vi "GageDeepAcquisition_ori.vi"() -> ()   [LabVIEW 2013]
uses:
  <vilib>/Analysis/NI_AALPro.lvlib
  <vilib>/Analysis/NI_AALBase.lvlib
  <vilib>/Utility/file.llb/Write To Spreadsheet File (DBL).vi
  <vilib>/Analysis/2dsp.llb/1D Cross Correlation (DBL).vi
panel:
  in  "하위 컷오프(MHz)":dbl
  in  "상위 컷오프(MHz)":dbl
  in  "시작":bool
  in  "Boolean":bool
  out "Path":path
  out "?":dbl[](graph)
  out "?":dbl[](graph)
  out "진행상황":string
  in  "crosscorr lacks":dbl=500.0
  out "Length":dbl=25000064.0
  out "?":dbl[](graph)
  in  "Trigger":T1={"Slope"=0, "Level"=0, "Source"=0, "External Range"=2000, "External Coupling"=0, "External"=FALSE, "Disable"=FALSE, "External Impedance"=1} {"External Impedance" items=["50 Ohm", "HiZ"]; "External Coupling" items=["DC", "AC"]; "External Range" min=2000 max=10000 step=8000; "Slope" items=["Rising", "Falling"]; "Level" min=-100 max=100; "Source" min=0 max=64 step=1}
  in  "stop":bool
  out "Page Size":dbl=98304.0 min=4096.0 step=4096.0
  out "Status":string
  in  "Channels":T2(array[cluster])=[{"Coupling"=0, "Differential Input"=FALSE, "Direct-to-ADC"=FALSE, "Range"=2000, "Impedance"=50, "DC Offset"=0, "Filter"=0}, {"Coupling"=0, "Differential Input"=FALSE, "Direct-to-ADC"=FALSE, "Range"=2000, "Impedance"=50, "DC Offset"=0, "Filter"=0}] {"Impedance" min=50 max=1000000 step=999950; "Coupling" items=["DC", "AC"]}
  in  "Acquisition":T3={"Sample Rate"=25000000.0, "Mode"=2, "Depth"=25000064.0, "Segment Size"=25000064.0, "Trigger Timeout"=1000000.0, "Trigger Holdoff"=0.0, "Trigger Delay"=0.0, "Clock mode"=enum."Internal"} {"Segment Size" min=256.0 step=128.0; "Trigger Delay" min=0.0 step=128.0; "Trigger Holdoff" min=0.0 step=128.0; "Depth" min=256.0 step=128.0; "Mode" items=["Single", "Dual", "Quad", "Octal"]}
  in  "Pages":i32=50 min=1 max=4000000 step=1
  out "System Name":string
  out "Channel Count":u16
  out "Board Count":u16
  in  "Start Point":dbl
  out "System Count":i32
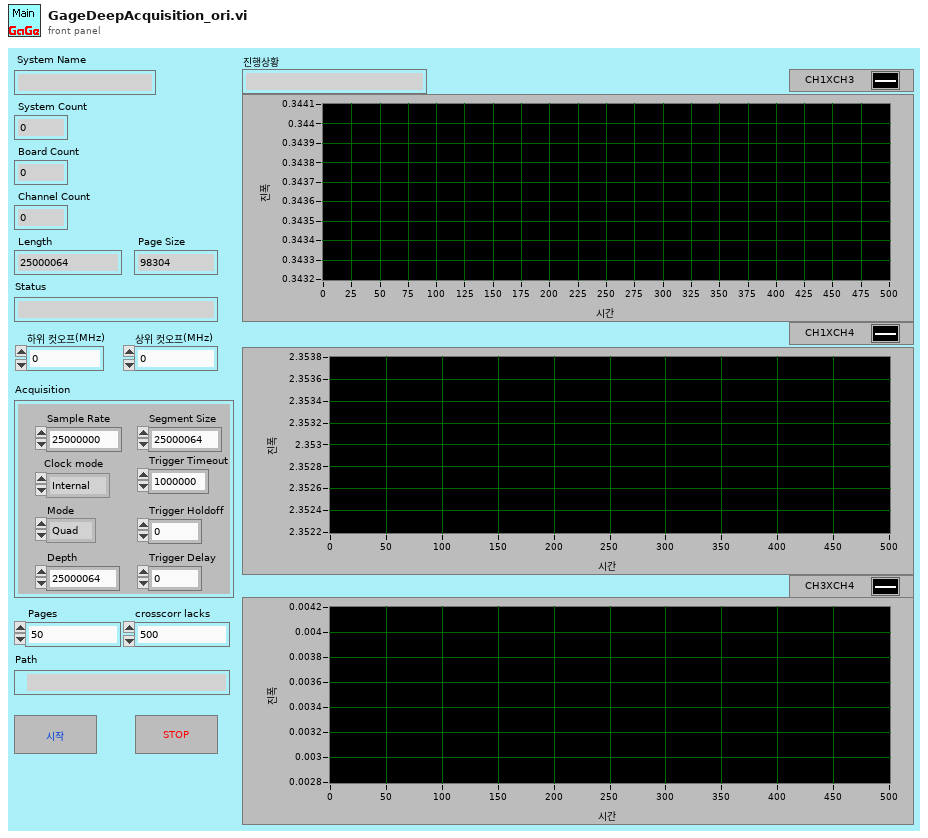
[diagram p1: front panel]
types:
  T1 = cluster{"Slope":u16, "Level":i32, "Source":i32, "External Range":u32, "External Coupling":u16, "External":bool, "Disable":bool, "External Impedance":u16}
  T2 = cluster{"Coupling":u16, "Differential Input":bool, "Direct-to-ADC":bool, "Range":u32, "Impedance":u32, "DC Offset":i32, "Filter":i32}[]
  T3 = cluster{"Sample Rate":dbl, "Mode":u16, "Depth":dbl, "Segment Size":dbl, "Trigger Timeout":dbl, "Trigger Holdoff":dbl, "Trigger Delay":dbl, "Clock mode":enum16{"Internal", "External", "Reference"}}
  T4 = cluster{"Handle":u32, "Sample size":u32, "Resolution":i32, "Offset":i32, "Channels":u32, "Boards":u32}
  T5 = cluster{"Coupling":u16, "Differential Input":bool, "Direct-to-ADC":bool, "Range":u32, "Impedance":u32, "DC Offset":i32, "Filter":i32}
  T6 = cluster{string, "Differential Input":bool, "Direct-to-ADC":bool, "Range":u32, "Impedance":u32, "DC Offset":i32, "Filter":i32}
  T7 = cluster{"RingText.Text":string, "Level":i32, "Source":i32, "External Range":u32, "RingText.Text":string, "External":bool, "Disable":bool, "RingText.Text":string}
  T8 = cluster{"Sample Rate":dbl, "Clock mode":enum16{"Internal", "External", "Reference"}, "RingText.Text":string, "Depth":dbl, "Segment Size":dbl, "Trigger Timeout":dbl, "Trigger Holdoff":dbl, "Trigger Delay":dbl}
  T9 = cluster{"RingText.Text":string, "Level":i32, "Source":i32, "External Range":u32, "RingText.Text":string, "External":bool, "Disable":bool, "RingText.Text":string}[]
  T10 = cluster{"Handle":u32, "Sample Size":u32, "Resolution":i32, "Offset":i32, "Channels":u32, "Boards":u32}
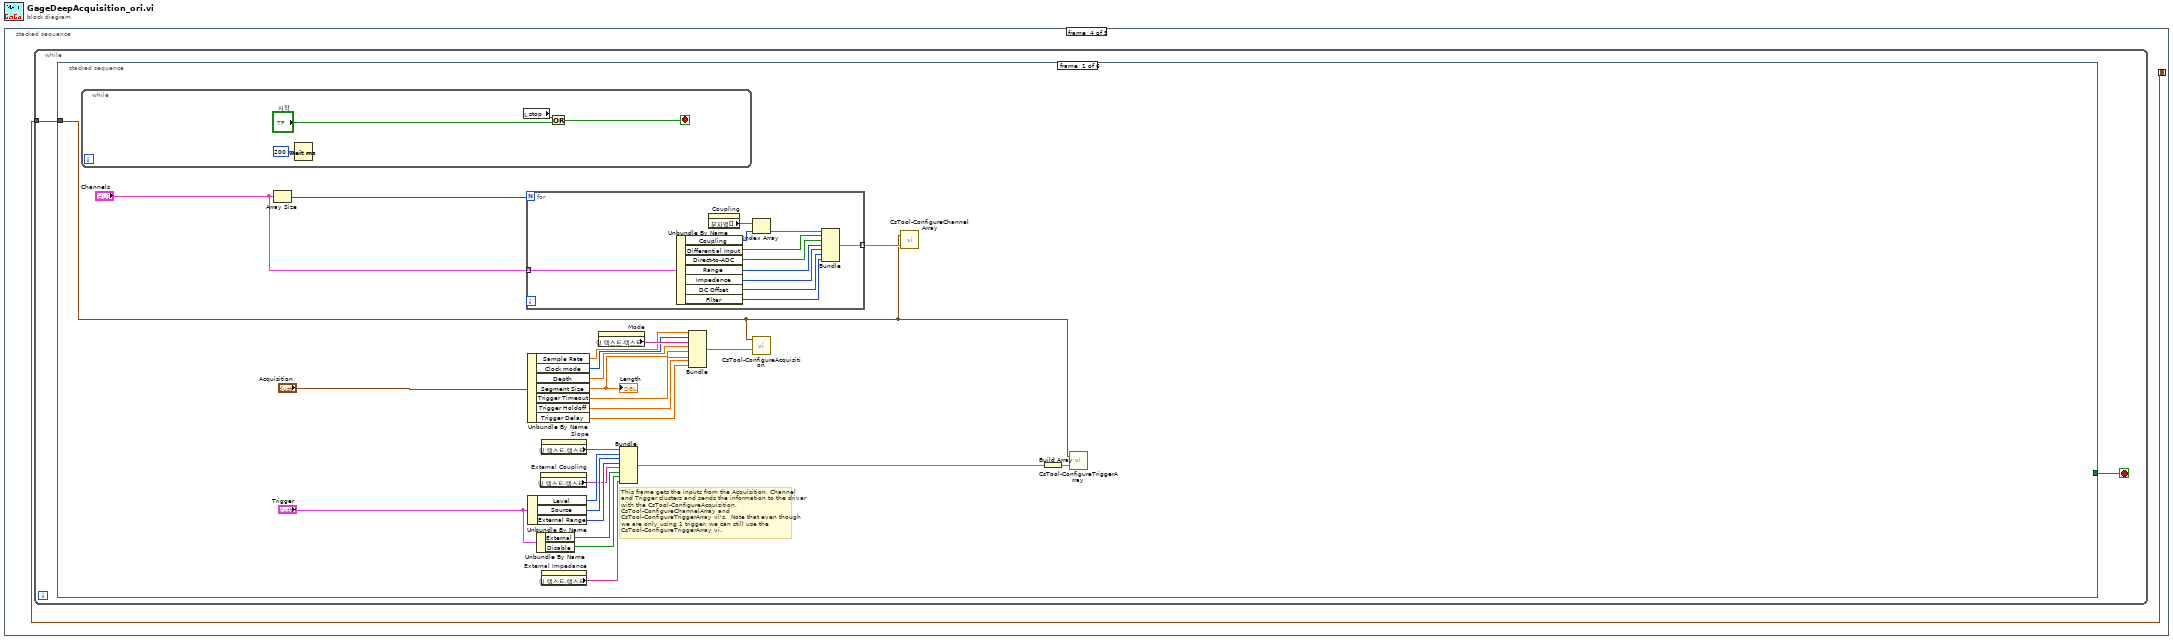
[diagram p0: block diagram]
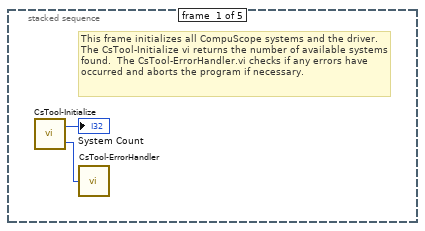
[diagram p2: hidden frame]
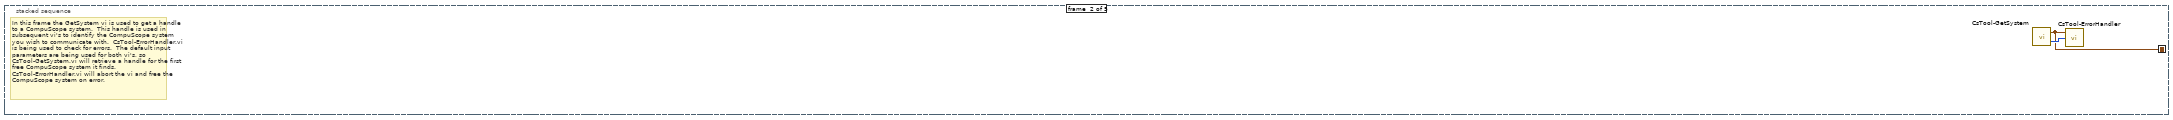
[diagram p3: hidden frame]
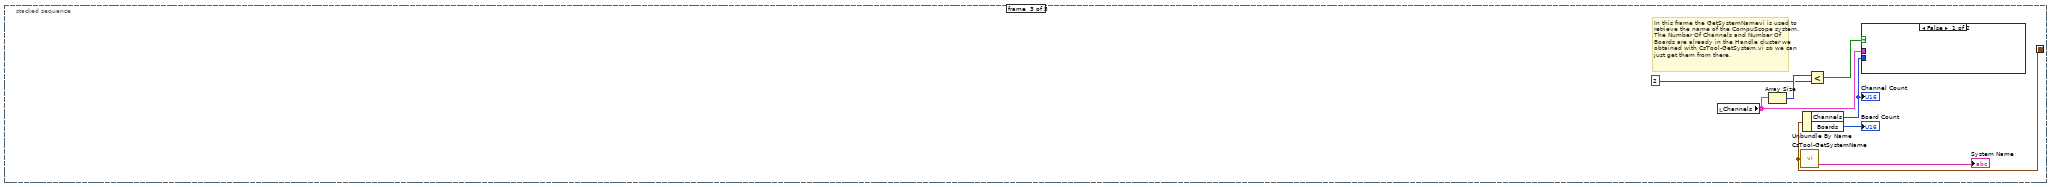
[diagram p4: hidden frame]
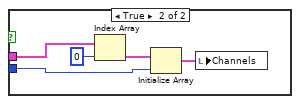
[diagram p5: hidden frame]
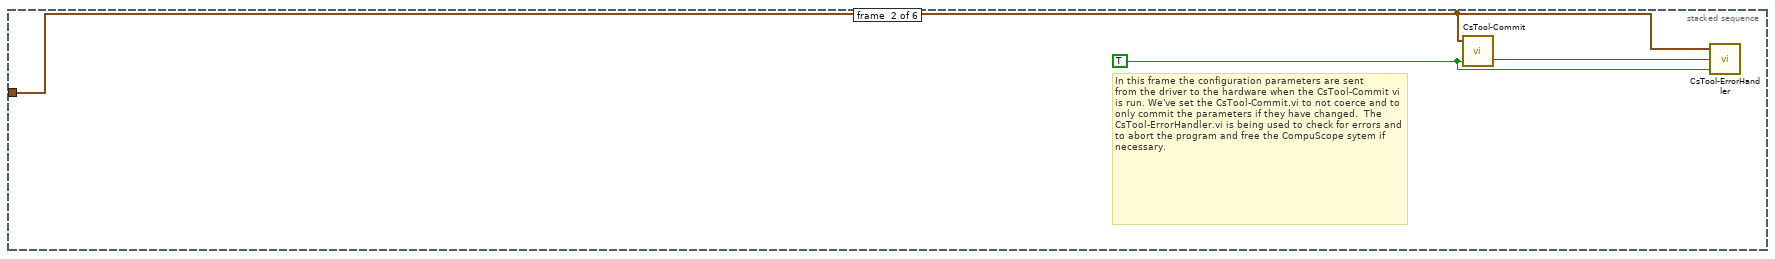
[diagram p6: hidden frame]
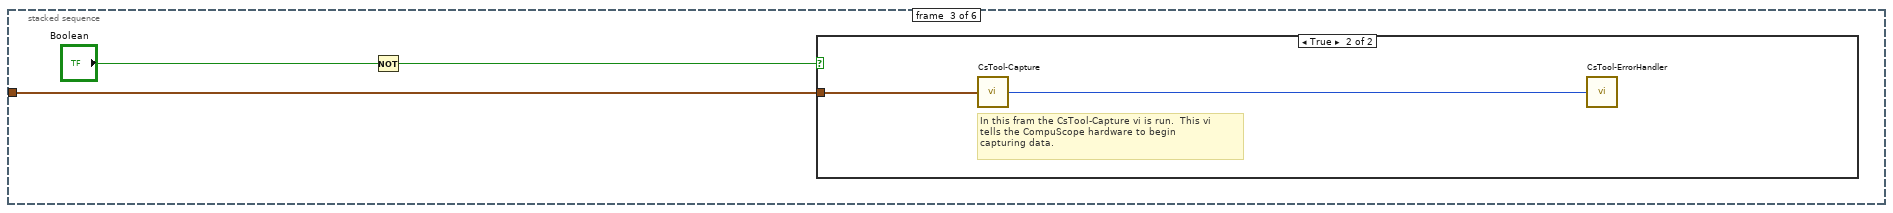
[diagram p7: hidden frame]
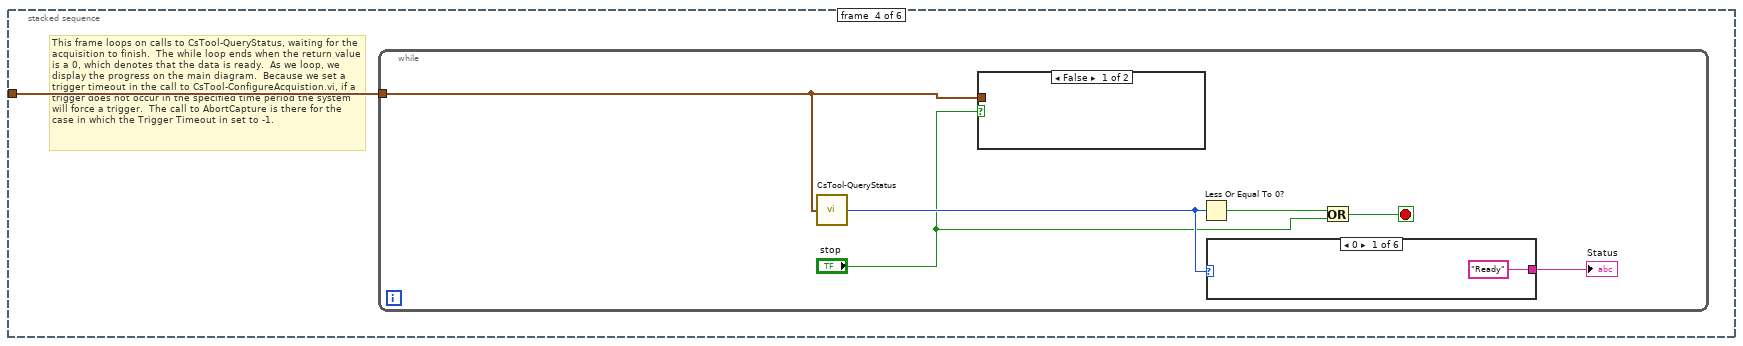
[diagram p9: hidden frame]
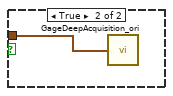
[diagram p10: hidden frame]
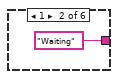
[diagram p11: hidden frame]
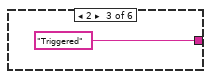
[diagram p12: hidden frame]
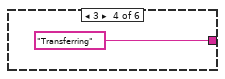
[diagram p13: hidden frame]
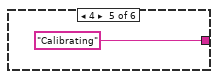
[diagram p14: hidden frame]
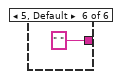
[diagram p15: hidden frame]
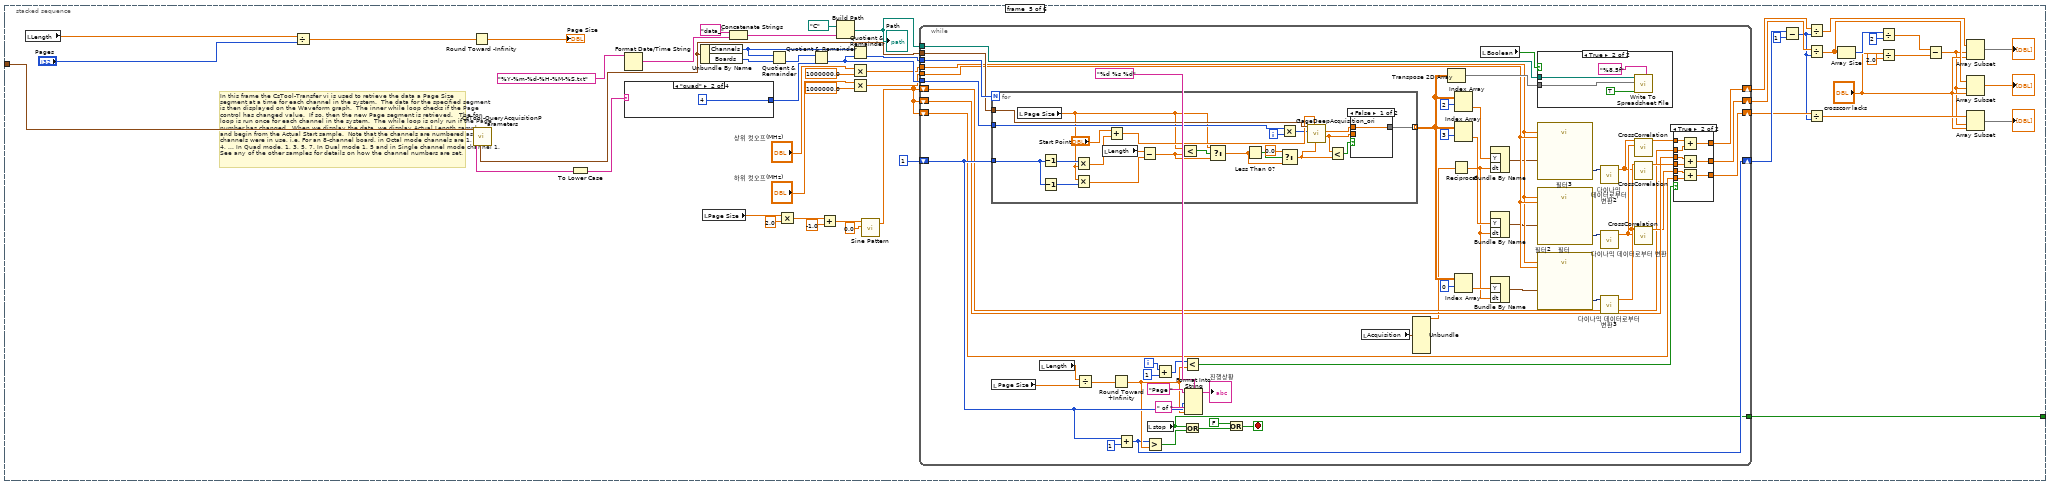
[diagram p16: hidden frame]
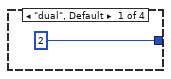
[diagram p17: hidden frame]
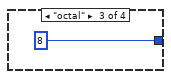
[diagram p18: hidden frame]
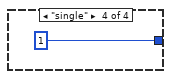
[diagram p19: hidden frame]
diagram:
  n1 = stacked-sequence {
    seq-local: [_ w3 _ _ _] -> [_ _ w11 w18 w249]
    frame #0 {
      # "This frame initializes all CompuScope systems and the driver.\nThe CsTool-Initialize vi returns the number of available systems found.  The CsTool-ErrorHandler.vi checks if any errors have occurred and aborts the program if necessary."
      n2 = call <userlib>:"CsTool-Initialize.vi"() -> ("Error Code"=w2:i32, "Number Of Systems"=→"System Count":i32)
      n3 = call <userlib>:"CsTool-ErrorHandler.vi"("Error Code"=w2) -> ()  [unwired: 2 in, 1 out]
    }
    frame #1 {
      # "In this frame the GetSystem vi is used to get a handle \nto a CompuScope system.  This handle is used in \nsubsequent vi's to identify the CompuScope system \nyou wish to communicate with.  CsTool-ErrorHandler.vi is being used to check for errors.  The default input parameters are being used for both vi's, so CsTool-GetSystem.vi will retrieve a handle for the first free CompuScope system it finds.  CsTool-ErrorHandler.vi will abort the vi and free the CompuScope system on error."
      n4 = call <userlib>:"CsTool-GetSystem.vi"() -> ("Error Code"=w4:i32, "Handle Cluster"=w3:T4)  [unwired: 4 in]
      n5 = call <userlib>:"CsTool-ErrorHandler.vi"("Error Code"=w4, "Handle Cluster"=w3) -> ()  [unwired: 1 in, 1 out]
    }
    frame #2 {
      # "In this frame the GetSystemNamevi is used to\nretrieve the name of the CompuScope system. The Number Of Channels and Number Of Boards are already in the Handle cluster we obtained with CsTool-GetSystem.vi so we can just get them from there."
      n6 = local read "Channels"() -> (w7:T2)
      n7 = Array Size(array=w7) -> (size(s)=w8:i32)
      n8 = call <userlib>:"CsTool-GetSystemName.vi"("Handle Cluster"=w11) -> ("System Name"=→"System Name":string)  [unwired: 1 out]
      n9 = Unbundle By Name(w11) -> ("Channels"=w10:u32, "Boards"=→"Board Count":u32)
      "Channel Count" <- w10
      n10 = Less?(x=w8, y=2) -> (x < y?=w9:bool)
      n11 = case shown="False" w9 {
        tunnel: w7 -> [_ w15]
        tunnel: w10 -> [_ w13]
        frame False {
        }
        frame True {
          n12 = Index Array(array=w15, index=0) -> (element=w14:T5)
          n13 = Initialize Array(w14, w13) -> (w16:T2)
          n14 = local write "Channels"(w16) -> ()
        }
      }
    }
    frame #3 {
      n15 = while {
        tunnel: w18 -> [w20]
        stop <- w19 stop-if-true
        n16 = stacked-sequence {
          tunnel: w20 -> [w39 w61 w66 w69 w135 _]
          tunnel: [_ _ _ _ w91 _] -> w19
          frame #0 {
            # "This frame gets the inputs from the Acquisition, Channel and Trigger clusters and sends the information to the driver with the CsTool-ConfigureAcquisition, CsTool-ConfigureChannelArray and CsTool-ConfigureTriggerArray vi's.  Note that even though we are only using 1 trigger, we can still use the CsTool-ConfigureTriggerArray vi."
            n17 = while {
              stop <- w46 stop-if-true
              n18 = Wait (ms)(milliseconds to wait=u32 200 ("대기 시간(ms)")) -> ()  [unwired: 1 out]
              n19 = local read "stop"() -> (w48:bool)
              n20 = Or(x=w48, y="시작") -> (x .or. y?=w46:bool)
            }
            n21 = Array Size(array="Channels") -> (size(s)=w42:i32)
            n22 = for {
              N: w42 -> [_]
              tunnel: "Channels" -> [w56] mode=indexing
              tunnel: [w57] -> w40 mode=indexing
              n23 = Unbundle By Name(w56) -> ("Coupling"=w60:u16, "Differential Input"=w55:bool, "Direct-to-ADC"=w54:bool, "Range"=w53:u32, "Impedance"=w52:u32, "DC Offset"=w51:i32, "Filter"=w50:i32)
              n24 = property on="Coupling" class="Ring (strict)"() -> ("문자열[]"=w59:string[])  [unwired: 2 in, 2 out]
              n25 = Index Array(array=w59, index=w60) -> (element=w58:string)
              n26 = Bundle(w58, "Differential Input"=w55, "Direct-to-ADC"=w54, "Range"=w53, "Impedance"=w52, "DC Offset"=w51, "Filter"=w50) -> (w57:T6)  [unwired: 1 in]
            }
            n27 = Unbundle By Name("Acquisition") -> ("Sample Rate"=w22:dbl, "Clock mode"=w23:enum16{"Internal", "External", "Reference"}, "Depth"=w45:dbl, "Segment Size"=w21:dbl, "Trigger Timeout"=w28:dbl, "Trigger Holdoff"=w27:dbl, "Trigger Delay"=w26:dbl)
            "Length" <- w21
            n28 = Unbundle By Name("Trigger") -> ("Level"=w37:i32, "Source"=w35:i32, "External Range"=w34:u32)
            n29 = Unbundle By Name("Trigger") -> ("External"=w36:bool, "Disable"=w33:bool)
            n30 = property on="External Coupling" class="Ring (strict)"() -> ("링 텍스트.텍스트"=w30:string)  [unwired: 2 in, 2 out]
            n31 = property on="Slope" class="Ring (strict)"() -> ("링 텍스트.텍스트"=w31:string)  [unwired: 2 in, 2 out]
            n32 = property on="External Impedance" class="Ring (strict)"() -> ("링 텍스트.텍스트"=w29:string)  [unwired: 2 in, 2 out]
            n33 = property on="Mode" class="Ring (strict)"() -> ("링 텍스트.텍스트"=w44:string)  [unwired: 2 in, 2 out]
            n34 = Bundle("RingText.Text"=w31, "Level"=w37, "Source"=w35, "External Range"=w34, "RingText.Text"=w30, "External"=w36, "Disable"=w33, "RingText.Text"=w29) -> (w25:T7)  [unwired: 1 in]
            n35 = Bundle("Sample Rate"=w22, "Clock mode"=w23, "RingText.Text"=w44, "Depth"=w45, "Segment Size"=w21, "Trigger Timeout"=w28, "Trigger Holdoff"=w27, "Trigger Delay"=w26) -> (w43:T8)  [unwired: 1 in]
            n36 = call <userlib>:"CsTool-ConfigureAcquisition.vi"("Handle Cluster"=w39, "Acquisition"=w43) -> ()  [unwired: 3 in, 1 out]
            n37 = call <userlib>:"CsTool-ConfigureChannelArray.vi"("Channels"=w40, "Handle Cluster"=w39) -> ()  [unwired: 1 out]
            n38 = Build Array(w25) -> (w24:T9)
            n39 = call <userlib>:"CsTool-ConfigureTriggerArray.vi"("Triggers"=w24, "Handle Cluster"=w39) -> ()  [unwired: 1 out]
          }
          frame #1 {
            w62 = TRUE
            # "In this frame the configuration parameters are sent\nfrom the driver to the hardware when the CsTool-Commit vi \nis run. We've set the CsTool-Commit.vi to not coerce and to\nonly commit the parameters if they have changed.  The CsTool-ErrorHandler.vi is being used to check for errors and to abort the program and free the CompuScope sytem if necessary."
            n40 = call <userlib>:"CsTool-Commit.vi"("OnlyOnChange (t)"=w62, "Handle Cluster"=w61) -> ("Error Code"=w63:i32)  [unwired: 1 in, 1 out]
            n41 = call <userlib>:"CsTool-ErrorHandler.vi"("StopOnError (true)"=w62, "Error Code"=w63, "Handle Cluster"=w61) -> ()  [unwired: 1 out]
          }
          frame #2 {
            n42 = Not(x="Boolean") -> (.not. x?=w65:bool)
            n43 = case shown="True" w65 {
              tunnel: w66 -> [_ w67]
              frame False {
              }
              frame True {
                # "In this fram the CsTool-Capture vi is run.  This vi\ntells the CompuScope hardware to begin\ncapturing data."
                n44 = call <userlib>:"CsTool-Capture.vi"("Handle Cluster"=w67) -> ("Error Code"=w68:i32)
                n45 = call <userlib>:"CsTool-ErrorHandler.vi"("Error Code"=w68) -> ()  [unwired: 2 in, 1 out]
              }
            }
          }
          frame #3 {
            # "This frame loops on calls to CsTool-QueryStatus, waiting for the acquisition to finish.  The while loop ends when the return value is a 0, which denotes that the data is ready.  As we loop, we display the progress on the main diagram.  Because we set a trigger timeout in the call to CsTool-ConfigureAcquistion.vi, if a trigger does not occur in the specified time period the system will force a trigger.  The call to AbortCapture is there for the case in which the Trigger Timeout in set to -1."
            n46 = while {
              tunnel: w69 -> [w71]
              stop <- w72 stop-if-true
              n47 = call <userlib>:"CsTool-QueryStatus.vi"("Handle Cluster"=w71) -> ("Status"=w75:i32)
              n48 = case shown="False" "stop" {
                tunnel: w71 -> [_ w76]
                frame False {
                }
                frame True {
                  n49 = call "GageDeepAcquisition_ori.vi"("Handle Cluster"=w76) -> ()  [unwired: 1 out]
                }
              }
              n50 = Less Or Equal To 0?(x=w75) -> (x <= 0?=w73:bool)
              n51 = case shown="0" w75 {
                tunnel: ["Ready" "Waiting" "Triggered" "Transferring" "Calibrating" " "] -> w74
                frame 0 {
                }
                frame 1 {
                }
                frame 2 {
                }
                frame 3 {
                }
                frame 4 {
                }
                frame 5, Default {
                }
              }
              "Status" <- w74
              n52 = Or(x=w73, y="stop") -> (x .or. y?=w72:bool)
            }
          }
          frame #4 {
            # "In this frame the CsTool-Transfer vi is used to retrieve the data a Page Size \nsegment at a time for each channel in the system.  The data for the specified segment is then displayed on the Waveform graph.  The inner while loop checks if the Page control has changed value.  If so, then the new Page segment is retrieved.   The for loop is run once for each channel in the system.  The while loop is only run if the Page number has changed.  When we display the data, we display Actual Length samples and begin from the Actual Start sample.  Note that the channels are numbered as if all channels were in use, i.e. For an 8-channel board, in Octal mode channels are 1, 2, 3, 4, ... In Quad mode, 1, 3, 5, 7. In Dual mode 1, 5 and in Single channel mode channel 1.  See any of the other samples for details on how the channel numbers are set."
            n53 = local read "Length"() -> (w118:dbl)
            n54 = Divide(x=w118, y="Pages") -> (x/y=w116:dbl)
            n55 = Round Toward -Infinity(1:w116) -> (0:→"Page Size":dbl)
            n56 = call <userlib>:"CsTool-QueryAcquisitionParameters.vi"("Handle Cluster"=w135) -> ("Output Handle Cluster"=w134:T10, "Mode"=w133:string)  [unwired: 9 out]
            n57 = To Lower Case(string=w133) -> (all lower case string=w132:string)
            n58 = Format Date/Time String(time format string (%c)="%Y-%m-%d-%H-%M-%S.txt" ("시간 포맷 문자열 (%c)")) -> (date/time string=w121:string)  [unwired: 2 in]
            n59 = case shown="\"quad\"" w132 {
              tunnel: [2 4 8 1] -> w130
              frame "dual", Default {
              }
              frame "quad" {
              }
              frame "octal" {
              }
              frame "single" {
              }
            }
            n60 = Unbundle By Name(w134) -> ("Channels"=w129:u32, "Boards"=w126:u32)
            n61 = local read "Page Size"() -> (w114:dbl)
            n62 = Concatenate Strings("data_", w121) -> (w122:string)
            n63 = Quotient & Remainder(x=w129, y=w126) -> (floor(x/y)=w131:u32)  [unwired: 1 out]
            n64 = Multiply(x=w114, y=2.0) -> (x*y=w112:dbl)
            n65 = Quotient & Remainder(x=w131, y=w130) -> (floor(x/y)=w128:u32)  [unwired: 1 out]
            n66 = Add(x=w112, y=-1.0) -> (x+y=w110:dbl)
            n67 = Build Path(base path=path "C:/", name or relative path=w122) -> (appended path=w92:path)
            "Path" <- w92
            n68 = Quotient & Remainder(x=w129, y=w128) -> (floor(x/y)=w127:u32)  [unwired: 1 out]
            n69 = Multiply(x="상위 컷오프(MHz)", y=1000000.0) -> (x*y=w88:dbl)
            n70 = Multiply(x="하위 컷오프(MHz)", y=1000000.0) -> (x*y=w85:dbl)
            n71 = call <vilib>:"Sine Pattern.vi"("amplitude"=0.0, "samples"=w110) -> ("Sinusoidal Pattern"=w101:dbl[])  [unwired: 2 in, 1 out]
            n72 = while {
              shift-right: [w169] -> w103
              shift-left: 1 -> [w183]
              tunnel: w134 -> [w187]
              tunnel: w127 -> [w191]
              tunnel: w128 -> [w190]
              tunnel: w92 -> [w180]
              shift-right: [w176] -> w120
              shift-left: w101 -> [w177]
              shift-right: [w163] -> w99
              shift-left: w101 -> [w161]
              shift-right: [w164] -> w100
              shift-left: w101 -> [w162]
              tunnel: [w160] -> w91
              tunnel: w88 -> [w155]
              tunnel: w85 -> [w156]
              i -> [w173]
              stop <- w196 stop-if-true
              n73 = for {
                N: w191 -> [_]
                tunnel: [w232] -> w158 mode=indexing
                tunnel: w187 -> [w235]
                tunnel: w183 -> [w218]
                tunnel: w190 -> [w215]
                i -> [w216]
                n74 = local read "Page Size"() -> (w213:dbl)
                n75 = Decrement(x=w218) -> (x-1=w230:i32)
                n76 = Decrement(x=w218) -> (x-1=w220:i32)
                n77 = Multiply(x=w230, y=w213) -> (x*y=w229:dbl)
                n78 = Multiply(x=w213, y=w220) -> (x*y=w226:dbl)
                n79 = local read "Length"() -> (w227:dbl)
                n80 = Add(x="Start Point", y=w229) -> (x+y=w228:dbl)
                n81 = Subtract(x=w227, y=w226) -> (x-y=w224:dbl)
                n82 = Less?(x=w213, y=w224) -> (x < y?=w225:bool)
                n83 = Select(t=w213, s=w225, f=w224) -> (s? t:f=w221:dbl)
                n84 = Less Than 0?(x=w221) -> (x < 0?=w223:bool)
                n85 = Multiply(x=w215, y=w216) -> (x*y=w214:u32)
                n86 = Select(t=0.0, s=w223, f=w221) -> (s? t:f=w219:dbl)
                n87 = call "GageDeepAcquisition_ori.vi"("Length (4096)"=w219, "Start (0)"=w228, "Channel (0)"=w214, "Handle Cluster"=w235) -> ("Actual Length"=w217:dbl, "Data in Volts"=w233:dbl[])  [unwired: 2 in, 2 out]
                n88 = Less?(x=w217, y=w219) -> (x < y?=w234:bool)
                n89 = case shown="False" w234 {
                  tunnel: w233 -> [w236 w239]
                  tunnel: [w236 w238] -> w232
                  tunnel: w217 -> [_ w237]
                  frame False {
                  }
                  frame True {
                    n90 = Array Subset(array=w239, length=w237) -> (w238:dbl[])  [unwired: 1 in]
                  }
                }
              }
              n91 = local read "Page Size"() -> (w189:dbl)
              n92 = local read "Length"() -> (w181:dbl)
              n93 = Divide(x=w181, y=w189) -> (x/y=w188:dbl)
              n94 = Round Toward +Infinity(x=w188) -> (ceil(x): smallest int >= x=w174:dbl)
              n95 = Add(x=w183, y=1) -> (x+y=w169:i32)
              n96 = Greater?(x=w169, y=w174) -> (0:w186:bool)
              n97 = local read "stop"() -> (w160:bool)
              n98 = Add(x=w173, y=1) -> (x+y=w171:i32)
              n99 = Less?(x=w171, y=w174) -> (x < y?=w170:bool)
              n100 = Or(x=w160, y=w186) -> (x .or. y?=w185:bool)
              n101 = Format Into String(format string="%d %s %d", initial string="Page ", w183, " of ", w174) -> (resulting string=→"진행상황":string)  [unwired: 1 in, 1 out]
              n102 = Or(x=FALSE, y=w185) -> (x .or. y?=w196:bool)
              n103 = local read "Acquisition"() -> (w147:T3)
              n104 = Unbundle(w147) -> ("Sample Rate"=w146:dbl)  [unwired: 7 out]
              n105 = Transpose 2D Array(2D array=w158) -> (transposed array=w179:dbl[][])
              n106 = Reciprocal(x=w146) -> (1/x=w143:dbl)
              n107 = Index Array(array=w158, index (row)=2 ("인덱스 (행)")) -> (element=w142:dbl[])  [unwired: 1 in]
              n108 = Index Array(array=w158, index (row)=3) -> (element=w145:dbl[])  [unwired: 1 in]
              n109 = Index Array(array=w158, index (row)=0 ("인덱스 (행)")) -> (element=w150:dbl[])  [unwired: 1 in]
              n110 = local read "Boolean"() -> (w159:bool)
              n111 = Bundle By Name("Y"=w142, "dt"=w143) -> (w141:waveform(dbl))  [unwired: 1 in]
              n112 = Bundle By Name("Y"=w145, "dt"=w143) -> (w144:waveform(dbl))  [unwired: 1 in]
              n113 = Bundle By Name("Y"=w150, "dt"=w143) -> (w149:waveform(dbl))  [unwired: 1 in]
              n114 = case shown="True" w159 {
                tunnel: w179 -> [_ w211]
                tunnel: w180 -> [_ w209]
                frame False {
                }
                frame True {
                  n115 = call-poly <vilib>:"Write To Spreadsheet File.vi"("format (%.3f)"="%8.5f", "append to file? (new file:F)"=TRUE, "2D data"=w211, "file path (dialog if empty)"=w209) -> ()  [unwired: 4 in, 1 out]
                }
              }
              n116 = call "필터3"("Lower Cut-Off"=w156, "Upper Cut-Off"=w155, "Signal"=w141) -> ("Filtered Signal"=w152:dynamicdata)  [unwired: 7 in, 1 out]
              n117 = call "필터"("Lower Cut-Off"=w156, "Upper Cut-Off"=w155, "Signal"=w144) -> ("Filtered Signal"=w157:dynamicdata)  [unwired: 7 in, 1 out]
              n118 = call "필터2"("Lower Cut-Off"=w156, "Upper Cut-Off"=w155, "Signal"=w149) -> ("Filtered Signal"=w148:dynamicdata)  [unwired: 7 in, 1 out]
              n119 = call "다이나믹 데이터로부터 변환2"("Dynamic Data Type"=w152) -> ("Array"=w151:dbl[])  [unwired: 3 in]
              n120 = call "다이나믹 데이터로부터 변환"("Dynamic Data Type"=w157) -> ("Array"=w153:dbl[])  [unwired: 3 in]
              n121 = call "다이나믹 데이터로부터 변환3"("Dynamic Data Type"=w148) -> ("Array"=w154:dbl[])  [unwired: 3 in]
              n122 = call-poly <vilib>:"CrossCorrelation.vi"("Y"=w153, "X"=w151) -> ("Rxy"=w165:dbl[])  [unwired: 8 in, 1 out]
              n123 = call-poly <vilib>:"CrossCorrelation.vi"("Y"=w151, "X"=w154) -> ("Rxy"=w175:dbl[])  [unwired: 8 in, 1 out]
              n124 = call-poly <vilib>:"CrossCorrelation.vi"("Y"=w153, "X"=w154) -> ("Rxy"=w166:dbl[])  [unwired: 8 in, 1 out]
              n125 = case shown="True" w170 {
                tunnel: w177 -> [w199 w208]
                tunnel: [w199 w207] -> w176
                tunnel: w175 -> [_ w206]
                tunnel: w166 -> [_ w205]
                tunnel: w165 -> [_ w204]
                tunnel: [w198 w203] -> w164
                tunnel: [w197 w202] -> w163
                tunnel: w162 -> [w198 w201]
                tunnel: w161 -> [w197 w200]
                frame False {
                }
                frame True {
                  n126 = Add(x=w204, y=w200) -> (x+y=w202:dbl[])
                  n127 = Add(x=w206, y=w208) -> (x+y=w207:dbl[])
                  n128 = Add(x=w205, y=w201) -> (x+y=w203:dbl[])
                }
              }
            }
            n129 = Subtract(x=w103, y=1) -> (x-y=w98:i32)
            n130 = Divide(x=w99, y=w98) -> (x/y=w96:dbl[])
            n131 = Divide(x=w120, y=w98) -> (x/y=w109:dbl[])
            n132 = Divide(x=w100, y=w98) -> (x/y=w97:dbl[])
            n133 = Array Size(array=w109) -> (size(s)=w108:i32)
            n134 = Divide(x=w108, y=2 ("크기")) -> (x/y=w105:dbl)
            n135 = Divide(x="crosscorr lacks", y=2.0) -> (x/y=w104:dbl)
            n136 = Subtract(x=w105, y=w104) -> (x-y=w94:dbl)
            n137 = Array Subset(array=w96, index=w94, length="crosscorr lacks") -> (→"?":dbl[])
            n138 = Array Subset(array=w109, index=w94, length="crosscorr lacks") -> (→"?":dbl[])
            n139 = Array Subset(array=w97, index=w94, length="crosscorr lacks") -> (→"?":dbl[])
          }
          frame #5 {
            n140 = local read "stop"() -> (w241:bool)
            n141 = Not(x=w241) -> (.not. x?=w240:bool)
            n142 = case shown="True" w240 {
              frame False {
              }
              frame True {
                n143 = local read "Boolean"() -> (w243:bool)
                n144 = Not(x=w243) -> (.not. x?=w242:bool)
                n145 = case shown="False" w242 {
                  frame False {
                    w244 = FALSE ("Boolean")
                    n146 = call "사용자에게 메시지 디스플레이2"("Enable"=TRUE) -> ()  [unwired: 9 in, 2 out]
                    n147 = local write "시작"(w244) -> ()
                    n148 = local write "Boolean"(w244) -> ()
                  }
                  frame True {
                    n149 = call "사용자에게 메시지 디스플레이"("Enable"=TRUE) -> ("확인"=w246:bool)  [unwired: 9 in, 1 out]
                    n150 = local write "시작"(w246) -> ()
                    n151 = local write "Boolean"(w246) -> ()
                  }
                }
              }
            }
          }
        }
      }
    }
    frame #4 {
      # "We set the Stop button (actually it's local variable) to False here so when the vi stops the Stop button will not stay depressed."
      # "In this frame, which is reached when the Stop\nis pressed, the CompuScope system is freed by\nrunning the CsTool-FreeSystem vi.  This frees \nany resources used by the system and makes \nit available for another program to use."
      n152 = local write "stop"(FALSE) -> ()
      n153 = call "GageDeepAcquisition_ori.vi"("Handle Cluster"=w249) -> ()  [unwired: 1 out]
    }
  }
